vi "Base Path.vi"() -> (2 "Base Path":path)   [LabVIEW 2024, in "Wordle Scorer.lvlib"]
uses:
  Wordle Scorer.lvlib
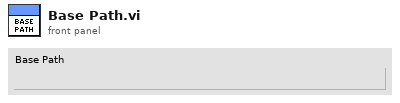
[diagram p1: front panel]
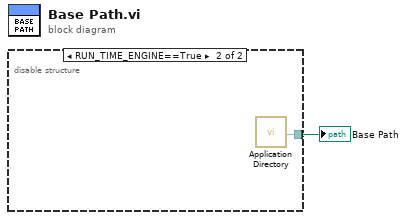
[diagram p0: block diagram]
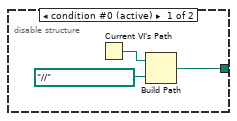
[diagram p2: hidden frame]
diagram:
  n1 = disable-structure shown="RUN_TIME_ENGINE==True" {
    disable-tunnel: [w2 w5] -> w1
    frame condition #0 (active) {
      n2 = Current VI's Path() -> (path=w3:path)
      n3 = Build Path(base path=w3, name or relative path=path "../../..") -> (appended path=w2:path)
    }
    frame condition #1 {
      n4 = call <vilib>:"Application Directory.vi"() -> ("Application Directory"=w5:path)
    }
  }
  "Base Path" <- w1
